vi "Add and Undo All.vi"(11 "Test Case In":refnum<class "Undo Redo Core.lvclass">) -> (0 "error out":errorcluster, 3 "Test Case Out":refnum<class "Undo Redo Core.lvclass">)   [LabVIEW 2021, in "Undo Redo Core.lvclass"]
uses:
  Undo Redo Core.lvclass
  <resource>/plugins/NIIconEditor/Controls/Undo Redo Action.ctl
  4993e8ee-a06a-463a-9684-69129f64d5ce.vi
panel:
  out "Undo Data":string[](array[string])
  out "Undo Variables":T1(array[cluster])
  out "Current State":string
  out "Current State Variables":T2
  out "Add Variables":T1(array[cluster])
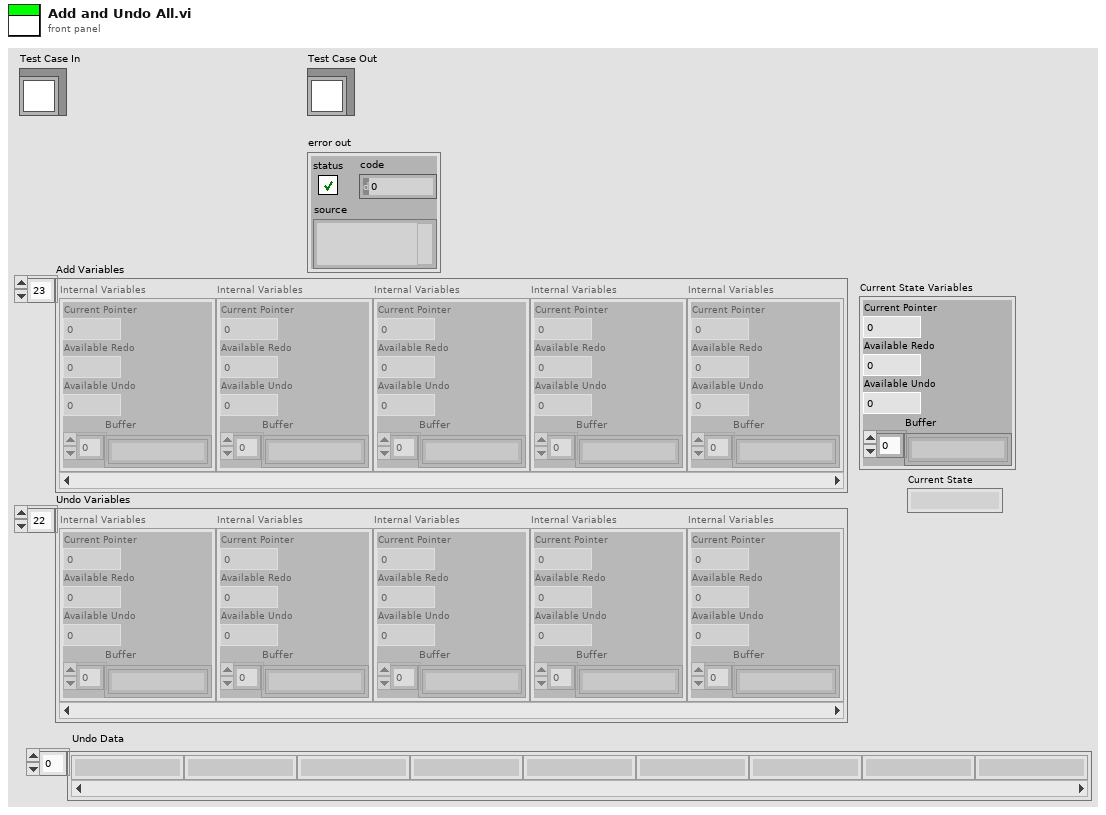
[diagram p1: front panel]
types:
  T1 = cluster{"Current Pointer":i32, "Available Redo":i32, "Available Undo":i32, "Buffer":string[]}[]
  T2 = cluster{"Current Pointer":i32, "Available Redo":i32, "Available Undo":i32, "Buffer":string[]}
  T3 = typedef "Undo Redo Action.ctl" = enum16{"Init", "Add", "Undo", "Redo", "Current State"}
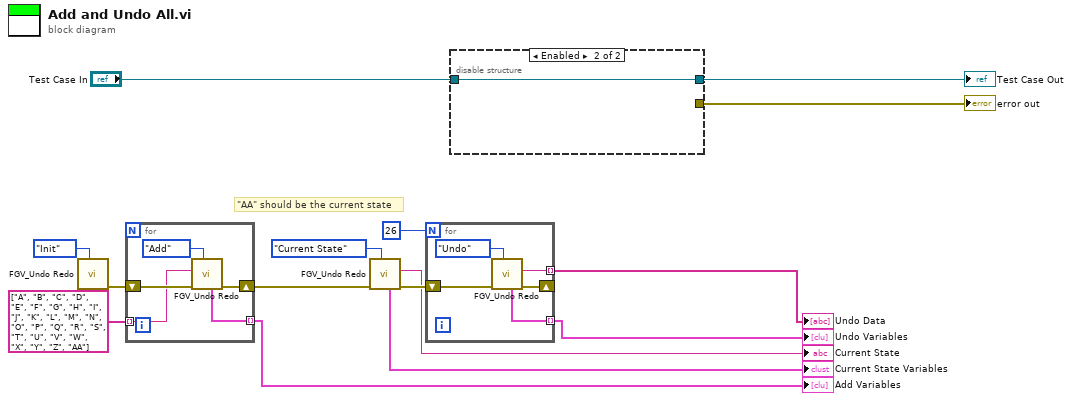
[diagram p0: block diagram]
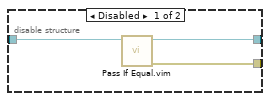
[diagram p2: hidden frame]
diagram:
  # "\"AA\" should be the current state"
  n1 = call <resource>:"FGV_Undo Redo.vi"("Action"=Undo_Redo_Action."Init") -> ("error out"=w14:errorcluster)  [unwired: 8 in, 2 out]
  n2 = for {
    tunnel: string[] ["A", "B", "C", "D", "E", "F", "G", "H", "I", "J", "K", "L", "M", "N", "O", "P", "Q", "R", "S", "T", "U", "V", "W", "X", "Y", "Z", "AA"] -> [w17] mode=indexing
    shift-right: [w19] -> w13
    shift-left: w14 -> [w20]
    tunnel: [w16] -> w7 mode=indexing
    n3 = call <resource>:"FGV_Undo Redo.vi"("Action"=Undo_Redo_Action."Add", "error in"=w20, "State in"=w17) -> ("error out"=w19:errorcluster, "Internal Variables"=w16:T2)  [unwired: 6 in, 1 out]
  }
  "Add Variables" <- w7
  n4 = call <resource>:"FGV_Undo Redo.vi"("Action"=Undo_Redo_Action."Current State", "error in"=w13) -> ("error out"=w12:errorcluster, "State out"=→"Current State":string, "Internal Variables"=→"Current State Variables":T2)  [unwired: 7 in]
  n5 = for {
    N: 26 -> [_]
    shift-right: [w24] -> _
    shift-left: w12 -> [w25]
    tunnel: [w22] -> w2 mode=indexing
    tunnel: [w21] -> w1 mode=indexing
    n6 = call <resource>:"FGV_Undo Redo.vi"("Action"=Undo_Redo_Action."Undo", "error in"=w25) -> ("error out"=w24:errorcluster, "State out"=w21:string, "Internal Variables"=w22:T2)  [unwired: 7 in]
  }
  "Undo Variables" <- w2
  "Undo Data" <- w1
  n7 = disable-structure shown="Enabled" {
    disable-tunnel: "Test Case In" -> [w27 w29]
    disable-tunnel: [w26 w29] -> w10
    disable-tunnel: [w28 _] -> w15
    frame Disabled {
      n8 = call "Pass If Equal.vim"("LUnit Test Case In"=w27) -> ("error out"=w28:errorcluster, "LUnit Test Case Out"=w26:refnum<class "Undo Redo Core.lvclass">)  [unwired: 9 in]
    }
    frame Enabled {
    }
  }
  "error out" <- w15
  "Test Case Out" <- w10
